vi "Write Shift Statistical Data To Excel.vi"(8 "Shift Timing":string="08:00:00-14:00:00", 9 "Shift Name":string="Shift 1", 10 "Shift End Date":string="27-Apr-2019", 11 "Statistical Shift Data":T1(array[cluster])=[{"PartName"="Part 1", "MeasurementNames"=["A", "B"], "Statistical Parameters"=[["Mean", "1.0", "6.0"], ["Standard Deviation", "2.0", "7.0"], ["Variance", "3.0", "8.0"], ["Cp", "4.0", "9.0"], ["Cpk", "5.0", "10.0"]]}, {"PartName"="Part 2", "MeasurementNames"=["C", "D"], "Statistical Parameters"=[["Mean", "1", "6"], ["Standard Deviation", "2", "7"], ["Variance", "3", "8"], ["Cp", "4", "9"], ["Cpk", "5", "10"]]}, {"PartName"="Part 3", "MeasurementNames"=["Ab", "Bc", "Cd"], "Statistical Parameters"=[["Mean", "10", "15", "20"], ["Standard Deviation", "11", "16", "21"], ["Variance", "12", "17", "22"], ["Cp", "13", "18", "23"], ["Cpk", "14", "19", "24"]]}]) -> (3 "Array":string[][](array[string]))   [LabVIEW 2019, in "DataLogger.lvclass"]
uses:
  DataLogger.lvclass
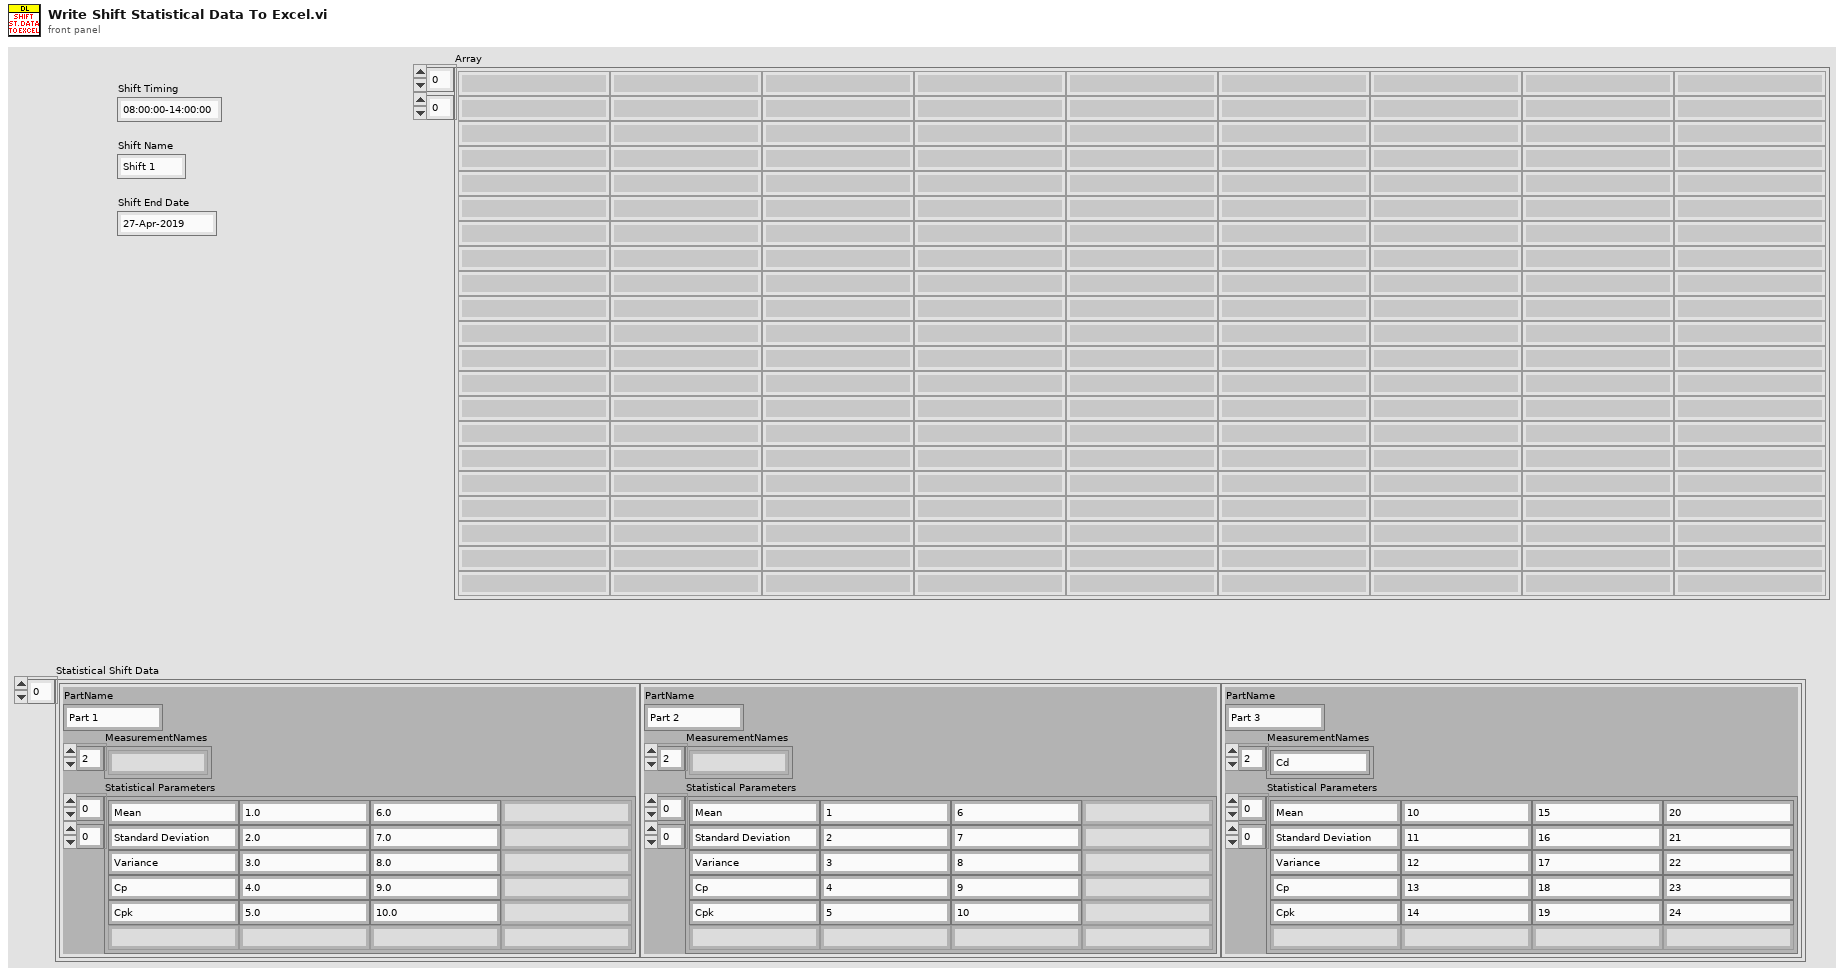
[diagram p1: front panel]
types:
  T1 = cluster{"PartName":string, "MeasurementNames":string[], "Statistical Parameters":string[][]}[]
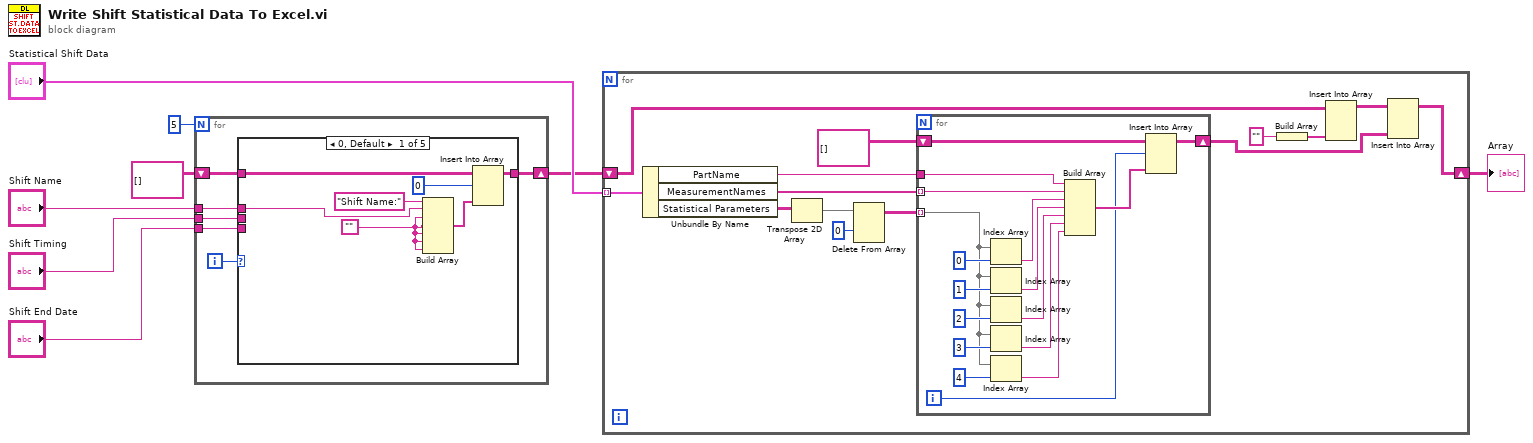
[diagram p0: block diagram]
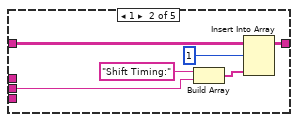
[diagram p2: hidden frame]
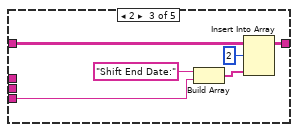
[diagram p3: hidden frame]
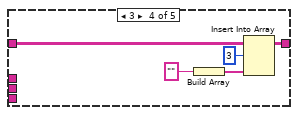
[diagram p4: hidden frame]
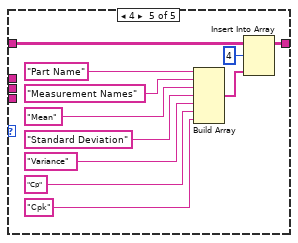
[diagram p5: hidden frame]
diagram:
  n1 = for {
    N: 5 -> [_]
    shift-right: [w11] -> w2
    shift-left: string[][] [] -> [w13]
    tunnel: "Shift Name" -> [w12]
    tunnel: "Shift Timing" -> [w10]
    tunnel: "Shift End Date" -> [w9]
    i -> [w14]
    n2 = case shown="0, Default" w14 {
      tunnel: w13 -> [w21 w27 w33 w38 w49]
      tunnel: w12 -> [w17 _ _ _ _]
      tunnel: [w16 w23 w29 w34 w45] -> w11
      tunnel: w10 -> [_ w22 _ _ _]
      tunnel: w9 -> [_ _ w28 _ _]
      frame 0, Default {
        w15 = ""
        n3 = Build Array("Shift Name:" ("new element/subarray"), w17, w15, w15, w15, w15, w15) -> (w19:string[])
        n4 = Insert Into Array(array=w21, index (row)=0 ("disabled index (col)"), new element=w19) -> (w16:string[][])  [unwired: 1 in]
      }
      frame 1 {
        n5 = Build Array("Shift Timing:" ("new element/subarray"), w22) -> (w25:string[])
        n6 = Insert Into Array(array=w27, index (row)=1 ("disabled index (col)"), new element=w25) -> (w23:string[][])  [unwired: 1 in]
      }
      frame 2 {
        n7 = Build Array("Shift End Date:" ("new element/subarray"), w28) -> (w31:string[])
        n8 = Insert Into Array(array=w33, index (row)=2 ("disabled index (col)"), new element=w31) -> (w29:string[][])  [unwired: 1 in]
      }
      frame 3 {
        n9 = Build Array("" ("new element/subarray")) -> (w36:string[])
        n10 = Insert Into Array(array=w38, index (row)=3 ("disabled index (col)"), new element=w36) -> (w34:string[][])  [unwired: 1 in]
      }
      frame 4 {
        n11 = Build Array("Part Name" ("new element/subarray"), "Measurement Names" ("element"), "Mean" ("element"), "Standard Deviation" ("element"), "Variance" ("element"), "Cp" ("element"), "Cpk" ("element")) -> (w47:string[])
        n12 = Insert Into Array(array=w49, index (row)=4 ("disabled index (col)"), new element=w47) -> (w45:string[][])  [unwired: 1 in]
      }
    }
  }
  n13 = for {
    tunnel: "Statistical Shift Data" -> [w63] mode=indexing
    shift-right: [w52] -> w1
    shift-left: w2 -> [w56]
    n14 = Unbundle By Name(w63) -> ("PartName"=w58:string, "MeasurementNames"=w59:string[], "Statistical Parameters"=w62:string[][])
    n15 = Transpose 2D Array(2D array=w62) -> (transposed array=w61:string[][])
    n16 = Delete From Array(array=w61, index (row)=0) -> (array with subset deleted=w51:string[][])  [unwired: 2 in, 1 out]
    n17 = for {
      tunnel: w59 -> [w74] mode=indexing
      tunnel: w58 -> [w75]
      tunnel: w51 -> [w73] mode=indexing
      shift-right: [w67] -> w50
      shift-left: string[][] [] -> [w66]
      i -> [w64]
      n18 = Index Array(array=w73, index=0) -> (element=w72:string)
      n19 = Index Array(array=w73, index=1) -> (element=w71:string)
      n20 = Index Array(array=w73, index=2) -> (element=w70:string)
      n21 = Index Array(array=w73, index=3) -> (element=w69:string)
      n22 = Index Array(array=w73, index=4) -> (element=w68:string)
      n23 = Build Array(w75, w74, w72, w71, w70, w69, w68) -> (w65:string[])
      n24 = Insert Into Array(array=w66, index (row)=w64, new element=w65) -> (w67:string[][])  [unwired: 1 in]
    }
    n25 = Build Array("" ("new element/subarray")) -> (w54:string[])
    n26 = Insert Into Array(array=w56, new element=w54) -> (w53:string[][])  [unwired: 2 in]
    n27 = Insert Into Array(array=w53, new element=w50) -> (w52:string[][])  [unwired: 2 in]
  }
  "Array" <- w1
